vi "inverse_kin6.vi"(5 "Reset":bool, 6 "Predicted \nHandle pose":T1, 7 "Parameters":T2={"Stimulus"={"Type"=enum."Off", "Phase"=0.0, "Amplitude"=[], "Injection point"=enum."Total pose", "Closed loop"=FALSE, "Offset"=[], "Tip -> world"=FALSE, "Frequency"=0.0, "Length"=0.0}, "Goal Filter A"={"Speedup max"=0.0, "Speedup thresh"=0.0, "Speedup nonlin"=0.0, "Filters"=[]}, "Mode controls"={"Hold"=FALSE, "Cancellation"=FALSE, "Goal filter"=FALSE, "Trigger"=FALSE}, "Manipulator type"=enum."Current piezo", "Manipulator calibration"={"Tool offsets"=[[0.0, 0.0, 36200.0]], "Handle light calibration"=[], "Base pivots"=[], "Output pivots"=[], "Length center"=0.0, "Workspace height"=[], "Workspace diameter"=[0.0, 0.0, 36200.0], "Stack travel"=400.0, "Saturation pos"=375.0, "Inverse filters"=[], "Strut length"=10000.0, "Tip light calibration"=[]}, "Network"={"Remote Host"="", "Send Status"=FALSE, "Send Port"=0, "Recv Commands"=FALSE, "Recv Port"=0}, "Goal Filter B"={"Speedup max"=0.0, "Speedup thresh"=0.0, "Speedup nonlin"=0.0, "Filters"=[]}, "Cancellation"={"KP"={"XY"=0.0, "Rxy"=0.0, "Z"=0.0, "Rz"=0.0}, "KI"=0.0, "KD"={"XY"=0.0, "Rxy"=0.0, "Z"=0.0, "Rz"=0.0}, "Max vel"=20.0, "Max acc"=0.001, "Int error limit"=3.0, "RCM gain"=0.0, "Bypass"=FALSE, "Degraded gain"=0.0}, "Transition time"=0.0, "Estimation"={"Link"={"Measure noise"=[], "Process noise"=[], "Alt process noise"=[], "Alt turnoff cycles"=20, "Innovation limit"=[], "Residue threshold"=0.0, "Enable"=FALSE}, "Handle"={"Measure noise"=[], "Process noise"=[], "State limits"=[], "Innovation limit"=[], "Prediction Lookahead"=0.0, "Enable"=FALSE}}} {"Transition time" format="%_3f"; "Cancellation"."Degraded gain" min=0 max=1 step=0.1 format="%#_3p"; "Cancellation"."RCM gain" min=0 max=1 step=0.1 format="%#_3p"; "Cancellation"."KD"."Rz" min=-1 max=1 step=0.01 format="%#_3p"; "Cancellation"."KD"."Rxy" min=-1 max=1 step=0.01 format="%#_3p"; "Cancellation"."KD"."Z" min=-1 max=1 step=0.01 format="%#_3p"; "Cancellation"."KD"."XY" min=-1 max=1 step=0.01 format="%#_3p"; "Cancellation"."KI" min=0 max=1 step=0.01 format="%#_3p"; "Cancellation"."KP"."Rz" min=-1 max=1 step=0.01 format="%#_3p"; "Cancellation"."KP"."Rxy" min=-1 max=1 step=0.01 format="%#_3p"; "Cancellation"."KP"."Z" min=-1 max=1 step=0.01 format="%#_3p"; "Cancellation"."KP"."XY" min=-1 max=1 step=0.01 format="%#_3p"; "Cancellation"."Max acc" format="%#_3p"; "Goal Filter B"."Filters"."V limit range" format="%_3p"; "Goal Filter B"."Filters"."V limit" format="%_3p"; "Goal Filter B"."Filters"."Upper Q" format="%_3f"; "Goal Filter B"."Filters"."Upper Fc" format="%_3p"; "Goal Filter B"."Filters"."Lower Q" format="%_3f"; "Goal Filter B"."Filters"."Scale factor" format="%_3f"; "Goal Filter B"."Filters"."Lower Fc" format="%_3p"; "Goal Filter B"."Speedup nonlin" format="%_3p"; "Goal Filter B"."Speedup thresh" format="%_3p"; "Goal Filter B"."Speedup max" format="%_3p"; "Manipulator calibration"."Tip light calibration" format="%#.1f"; "Manipulator calibration"."Strut length" format="%#_4p"; "Manipulator calibration"."Saturation pos" format="%#.1f"; "Manipulator calibration"."Stack travel" format="%#.1f"; "Manipulator calibration"."Length center" format="%#_4p"; "Manipulator calibration"."Output pivots" format="%#_6f"; "Manipulator calibration"."Base pivots" format="%#_6f"; "Manipulator calibration"."Handle light calibration" format="%#.1f"; "Goal Filter A"."Filters"."V limit range" format="%_3p"; "Goal Filter A"."Filters"."V limit" format="%_3p"; "Goal Filter A"."Filters"."Upper Q" format="%_3f"; "Goal Filter A"."Filters"."Upper Fc" format="%_3p"; "Goal Filter A"."Filters"."Lower Q" format="%_3f"; "Goal Filter A"."Filters"."Scale factor" format="%_3f"; "Goal Filter A"."Filters"."Lower Fc" format="%_3p"; "Goal Filter A"."Speedup nonlin" format="%_3p"; "Goal Filter A"."Speedup thresh" format="%_3p"; "Goal Filter A"."Speedup max" format="%_3p"; "Stimulus"."Length" min=0.0 max=100.0 step=100.0 format="%#_4p"; "Stimulus"."Frequency" min=0.0 step=100.0 format="%#_4g"; "Stimulus"."Offset" format="%#_3p"; "Stimulus"."Amplitude" format="%#_3p"; "Stimulus"."Phase" min=-180.0 max=360.0 step=100.0 format="%#.2f"}, 10 "Output pose":T1, 11 "Handle pose":T1) -> (2 "Link goal":sgl[](array[numeric]), 3 "Link position":sgl[](array[numeric]))   [LabVIEW 2014]
uses:
  <vilib>/Analysis/Matrix/Datatypes/RealMatrix.ctl
  testing/Micron params.ctl
  testing/stimulus.ctl
  testing/injection_point.ctl
  filtering/goal_loop_parms.ctl
  testing/mode_conrols.ctl
  testing/manipulator_cal.ctl
  asap/labview/testing/probe_calibration.ctl
  host/network_params.ctl
  sq_control_params.ctl
  decoupled_gain.ctl
  estimation_controls.ctl
  <vilib>/Analysis/baseanly.llb/Real A x B.vi
  <vilib>/Analysis/NI_AALBase.lvlib
  <vilib>/Analysis/Matrix/NI_Matrix.lvlib
panel:
  # "Find actual and goal link lengths"
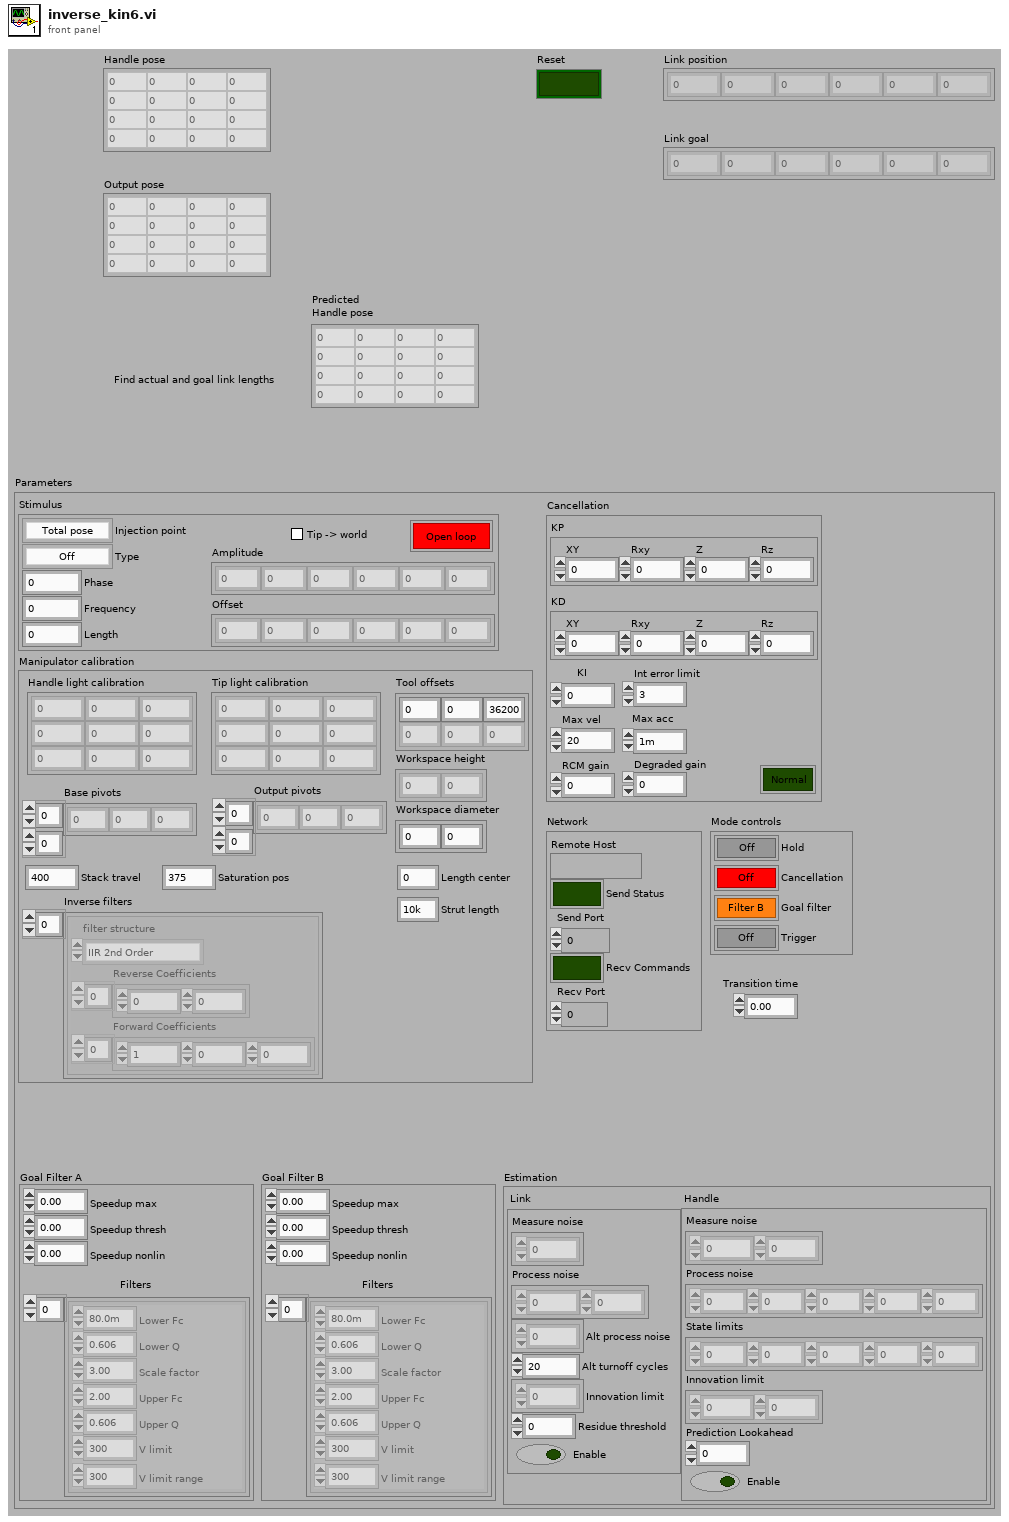
[diagram p1: front panel]
types:
  T1 = typedef "NI_Matrix.lvlib/RealMatrix.ctl" = dbl[][]
  T2 = typedef "Micron params.ctl" = cluster{"Stimulus":T3, "Goal Filter A":T5, "Mode controls":T6, "Manipulator type":enum16{"Current piezo", "Voltage piezo"}, "Manipulator calibration":T7, "Network":T9, "Goal Filter B":T5, "Cancellation":T10, "Transition time":sgl, "Estimation":T12}
  T3 = typedef "stimulus.ctl" = cluster{"Type":enum16{"Off", "Step", "Sine", "Triangle", "Arbitrary"}, "Phase":dbl, "Amplitude":sgl[], "Injection point":T4, "Closed loop":bool, "Offset":sgl[], "Tip -> world":bool, "Frequency":dbl, "Length":dbl}
  T4 = typedef "injection_point.ctl" = enum16{"Total pose", "V limiter", "Goal ", "Link position", "KF link position", "Inverse kin", "Link goal", "Link error", "Controller", "Output", "Drive", "Light"}
  T5 = typedef "goal_loop_parms.ctl" = cluster{"Speedup max":sgl, "Speedup thresh":sgl, "Speedup nonlin":sgl, "Filters":cluster{"Lower Fc":sgl, "Lower Q":sgl, "Scale factor":sgl, "Upper Fc":sgl, "Upper Q":sgl, "V limit":sgl, "V limit range":sgl}[]}
  T6 = typedef "mode_conrols.ctl" = cluster{"Hold":bool, "Cancellation":bool, "Goal filter":bool, "Trigger":bool}
  T7 = typedef "manipulator_cal.ctl" = cluster{"Tool offsets":sgl[][], "Handle light calibration":T8, "Base pivots":sgl[][], "Output pivots":sgl[][], "Length center":sgl, "Workspace height":sgl[], "Workspace diameter":sgl[], "Stack travel":sgl, "Saturation pos":sgl, "Inverse filters":cluster{"filter structure":enum32{"IIR 2nd Order", "IIR 4th Order"}, "Reverse Coefficients":dbl[], "Forward Coefficients":dbl[]}[], "Strut length":sgl, "Tip light calibration":T8}
  T8 = typedef "probe_calibration.ctl" = sgl[][]
  T9 = typedef "network_params.ctl" = cluster{"Remote Host":string, "Send Status":bool, "Send Port":u16, "Recv Commands":bool, "Recv Port":u16}
  T10 = typedef "sq_control_params.ctl" = cluster{"KP":T11, "KI":sgl, "KD":T11, "Max vel":sgl, "Max acc":sgl, "Int error limit":sgl, "RCM gain":sgl, "Bypass":bool, "Degraded gain":sgl}
  T11 = typedef "decoupled_gain.ctl" = cluster{"XY":sgl, "Rxy":sgl, "Z":sgl, "Rz":sgl}
  T12 = typedef "estimation_controls.ctl" = cluster{"Link":cluster{"Measure noise":dbl[], "Process noise":dbl[], "Alt process noise":dbl[], "Alt turnoff cycles":i32, "Innovation limit":dbl[], "Residue threshold":dbl, "Enable":bool}, "Handle":cluster{"Measure noise":dbl[], "Process noise":dbl[], "State limits":dbl[], "Innovation limit":dbl[], "Prediction Lookahead":sgl, "Enable":bool}}
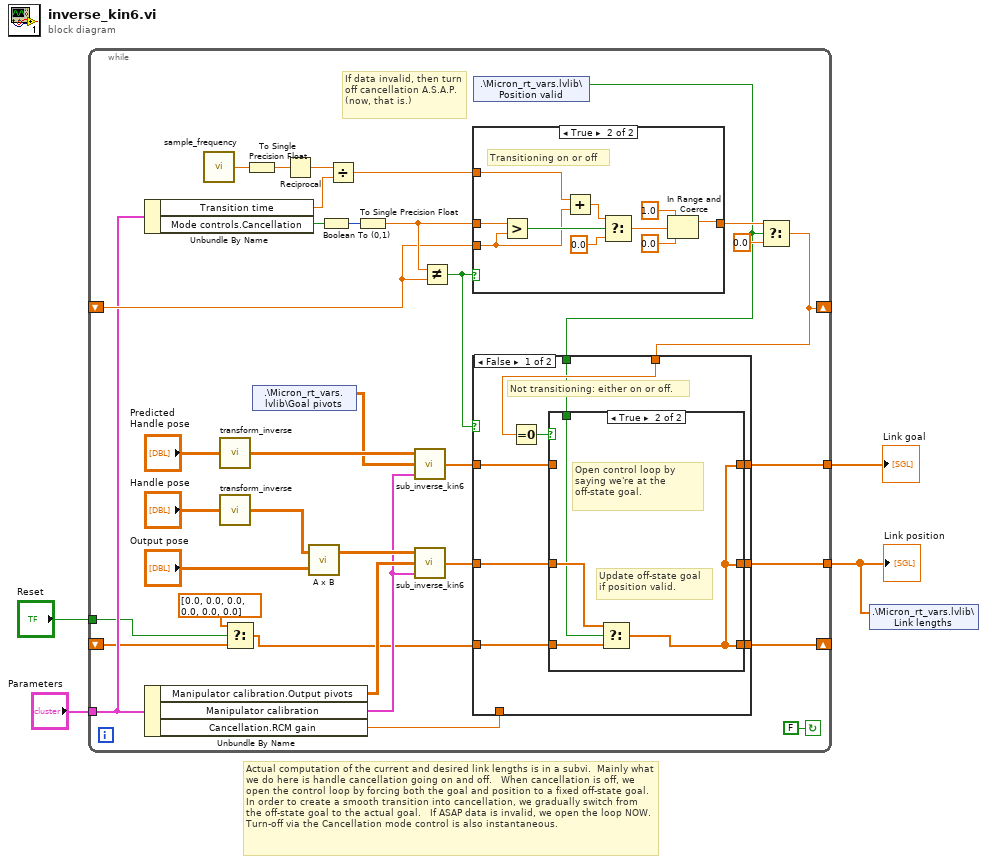
[diagram p0: block diagram]
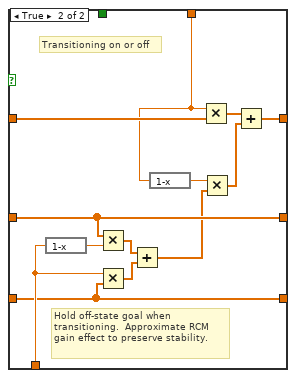
[diagram p3: hidden frame]
diagram:
  # "Actual computation of the current and desired link lengths is in a subvi.  Mainly what we do here is handle cancellation going on and off.   When cancellation is off, we open the control loop by forcing both the goal and position to a fixed off-state goal.   In order to create a smooth transition into cancellation, we gradually switch from the off-state goal to the actual goal.   If ASAP data is invalid, we open the loop NOW.   Turn-off via the Cancellation mode control is also instantaneous."
  n1 = while {
    shift-right: [w20] -> _
    shift-left: _ -> [w21]
    tunnel: "Parameters" -> [w19]
    shift-right: [w16] -> _
    shift-left: _ -> [w8]
    tunnel: [w15] -> w3
    tunnel: [w14] -> w2
    tunnel: "Reset" -> [w7]
    stop <- FALSE continue-if-true
    # "If data invalid, then turn off cancellation A.S.A.P. (now, that is.)"
    n2 = Unbundle By Name(w19) -> ("Transition time"=w29:sgl, "Mode controls.Cancellation"=w28:bool)
    n3 = Unbundle By Name(w19) -> ("Manipulator calibration.Output pivots"=w37:sgl[][], "Manipulator calibration"=w35:T7, "Cancellation.RCM gain"=w10:sgl)
    n4 = call "sample_frequency.vi"() -> ("Sample frequency"=w24:dbl)
    n5 = call "transform_inverse.vi"("Transform"="Predicted \nHandle pose") -> ("Inverse transform"=w36:T1)
    n6 = call "transform_inverse.vi"("Transform"="Handle pose") -> ("Inverse transform"=w13:T1)
    n7 = Select(t=sgl[] [0.0, 0.0, 0.0, 0.0, 0.0, 0.0], s=w7, f=w8) -> (s? t:f=w9:sgl[])
    n8 = To Single Precision Float(number=w24) -> (single precision float=w23:sgl)
    n9 = shared-variable ".\\Micron_rt_vars.lvlib\\Goal pivots"() -> (w34:sgl[][])  [unwired: 1 in, 1 out]
    n10 = Reciprocal(x=w23) -> (1/x=w31:sgl)
    n11 = call-poly <vilib>:"A x B.vi"("B"="Output pose", "A"=w13) -> ("A x B"=w39:T1)  [unwired: 1 out]
    n12 = Boolean To (0,1)(Boolean=w28) -> (0, 1=w33:i16)
    n13 = Divide(x=w31, y=w29) -> (x/y=w30:sgl)
    n14 = To Single Precision Float(number=w33) -> (single precision float=w32:sgl)
    n15 = call "sub_inverse_kin6.vi"("Manipulator calibration"=w35, "Output pivots"=w34, "Transform"=w36) -> ("Link lengths"=w27:sgl[])
    n16 = call "sub_inverse_kin6.vi"("Manipulator calibration"=w35, "Output pivots"=w37, "Transform"=w39) -> ("Link lengths"=w18:sgl[])
    n17 = Not Equal?(x=w32, y=w21) -> (x != y?=w17:bool)
    n18 = case shown="True" w17 {
      tunnel: w30 -> [_ w71]
      tunnel: w32 -> [w68 w73]
      tunnel: [w68 w72] -> w26
      tunnel: w21 -> [_ w70]
      frame False {
        # "Not transitioning, either on or off"
      }
      frame True {
        # "Transitioning on or off"
        n19 = Greater?(x=w73, y=w70) -> (0:w78:bool)
        n20 = Add(x=w71, y=w70) -> (x+y=w77:sgl)
        n21 = Select(t=w77, s=w78, f=sgl 0.0) -> (s? t:f=w76:sgl)
        n22 = In Range and Coerce(upper limit=sgl 1.0, x=w76, lower limit=sgl 0.0) -> (coerced(x)=w72:sgl)  [unwired: 1 out]
      }
    }
    n23 = shared-variable ".\\Micron_rt_vars.lvlib\\Position valid"() -> (w5:bool)  [unwired: 2 out]
    n24 = Select(t=w26, s=w5, f=sgl 0.0) -> (s? t:f=w20:sgl)
    n25 = case shown="False" w17 {
      tunnel: w27 -> [w46 w67]
      tunnel: w20 -> [w47 w63]
      tunnel: w18 -> [w44 w56]
      tunnel: [w40 w59] -> w16
      tunnel: w9 -> [w42 w59]
      tunnel: [w43 w56] -> w14
      tunnel: [w45 w62] -> w15
      tunnel: w5 -> [w41 _]
      tunnel: w10 -> [_ w60]
      frame False {
        # "Not transitioning: either on or off."
        n26 = Equal To 0?(x=w47) -> (x = 0?=w48:bool)
        n27 = case shown="True" w48 {
          tunnel: w46 -> [w50 _]
          tunnel: [w50 w51] -> w45
          tunnel: w44 -> [w49 w54]
          tunnel: [w49 w51] -> w43
          tunnel: w42 -> [_ w53]
          tunnel: w41 -> [_ w52]
          tunnel: [w49 w51] -> w40
          frame False {
            # "Update off-state goal"
            # "On: route signals through."
          }
          frame True {
            # "Update off-state goal\nif position valid."
            # "Open control loop by saying we're at the off-state goal."
            n28 = Select(t=w54, s=w52, f=w53) -> (s? t:f=w51:sgl[])
          }
        }
      }
      frame True {
        # "Hold off-state goal when transitioning.  Approximate RCM gain effect to preserve stability."
        # "Transitioning on or off"
        n29 = expression code="1-x"(w60) -> (w61:sgl)
        n30 = Multiply(x=w56, y=w61) -> (x*y=w58:sgl[])
        n31 = Multiply(x=w60, y=w59) -> (x*y=w57:sgl[])
        n32 = Add(x=w58, y=w57) -> (x+y=w55:sgl[])
        n33 = expression code="1-x"(w63) -> (w66:sgl)
        n34 = Multiply(x=w63, y=w67) -> (x*y=w65:sgl[])
        n35 = Multiply(x=w66, y=w55) -> (x*y=w64:sgl[])
        n36 = Add(x=w65, y=w64) -> (x+y=w62:sgl[])
      }
    }
  }
  "Link position" <- w2
  "Link goal" <- w3
  n37 = shared-variable ".\\Micron_rt_vars.lvlib\\Link lengths"(w2) -> ()  [unwired: 1 in, 1 out]
